vi "Constructor.vi"(7 "TimeZoneInfoId":string, 8 "error in":errorcluster, 9 "Value":timestamp, 10 "Name":string, 11 "DateTime in":refnum<class "DateTime.lvclass">) -> (0 "error out":errorcluster, 3 "DateTime out":refnum<class "DateTime.lvclass">)   [LabVIEW 2021, in "ProligentXMLGenerator.lvlib" / "DateTime.lvclass"]
uses:
  DateTime.lvclass
  DateTime.lvclass/DateTime.ctl
  Attribute/Attribute.lvclass
  C:/Projects/proligent-xml-generator-labview/src/ProligentXMLGenerator/Base/Attribute/Attribute.lvclass
  C:/Projects/proligent-xml-generator-labview/src/ProligentXMLGenerator/Base/DateTime/DateTime.lvclass
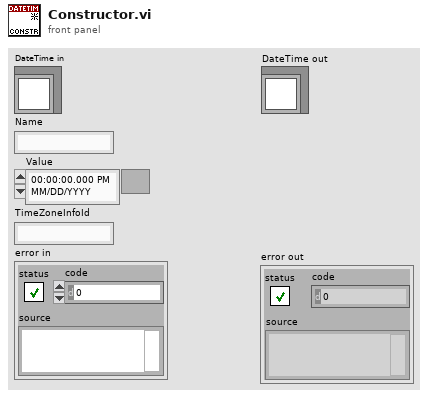
[diagram p1: front panel]
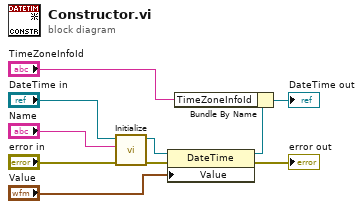
[diagram p0: block diagram]
diagram:
  n1 = call "Initialize.vi"("error in"="error in", "Name"="Name", "Attribute in"="DateTime in") -> ("error out"=w6:errorcluster, "Attribute out"=w5:refnum<class "DateTime.lvclass">)  [unwired: 7 in]
  n2 = property on="Property Node" class="DateTime"(reference=w5, error in=w6, "Value"="Value") -> (reference out=w3:refnum<class "DateTime.lvclass">, error out=→"error out":errorcluster)
  n3 = Bundle By Name(cluster=w3, "TimeZoneInfoId"="TimeZoneInfoId") -> (→"DateTime out":refnum<class "DateTime.lvclass">)
